vi "AttackerPenalty.vi"(6 "balls":T2[](array[typedef]), 8 "Opponent goalie":T1, 9 "Field Size in":T3, 10 "Numeric":i32, 11 "Robot in":T1) -> (3 "Robot out":T1)   [LabVIEW 2016]
uses:
  Core/AI Robot.ctl
  Core/Field Size.ctl
  Core/AI Ball.ctl
  <vilib>/Analysis/coordinate.llb/Angle Units.ctl
  <vilib>/Analysis/coordinate.llb/Absolute Angle Difference (scalar).vi
  <vilib>/Analysis/coordinate.llb/Wrap Angle (scalar).vi
  <vilib>/Analysis/coordinate.llb/Set Angle Unit.vi
  <vilib>/Analysis/NI_AAL_Angle.lvlib
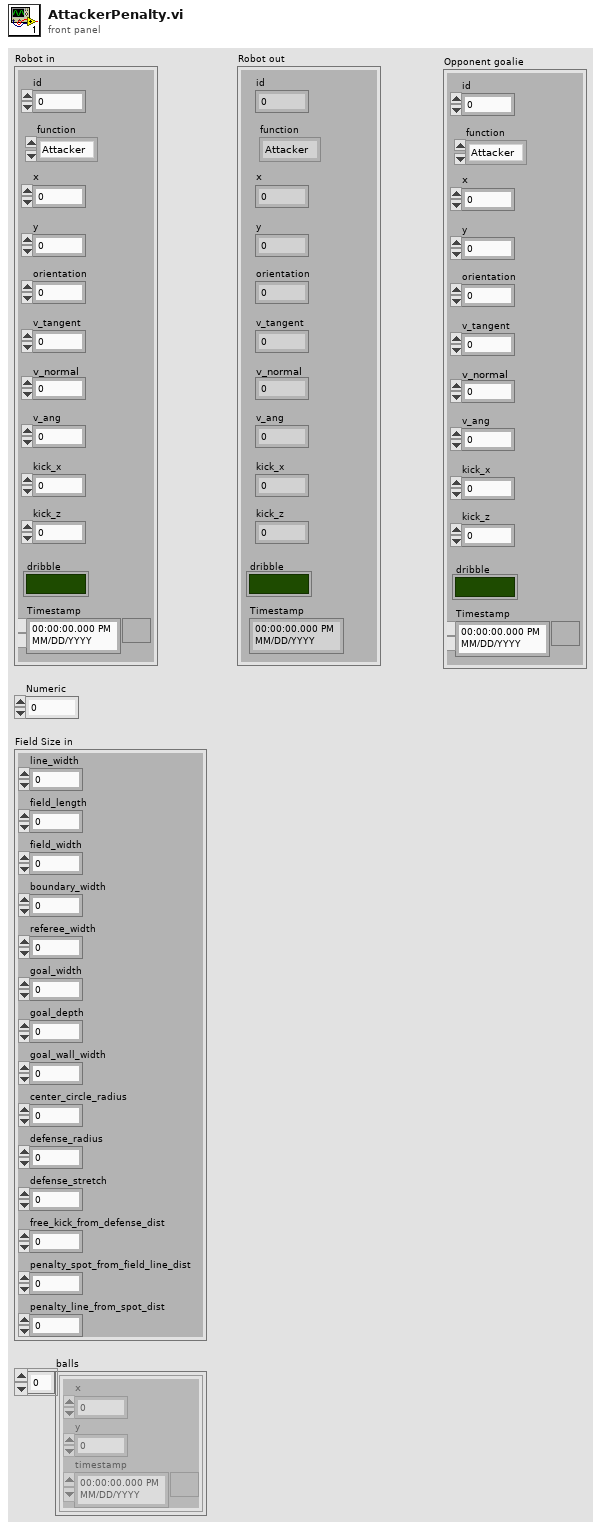
[diagram p1: front panel]
types:
  T1 = typedef "AI Robot.ctl" = cluster{"id":u32, "function":enum16{"Attacker", "Goalie", "Defender"}, "x":dbl, "y":dbl, "orientation":dbl, "v_tangent":dbl, "v_normal":dbl, "v_ang":dbl, "kick_x":dbl, "kick_z":dbl, "dribble":bool, "Timestamp":timestamp}
  T2 = typedef "AI Ball.ctl" = cluster{"x":dbl, "y":dbl, "timestamp":timestamp}
  T3 = typedef "Field Size.ctl" = cluster{"line_width":u32, "field_length":u32, "field_width":u32, "boundary_width":u32, "referee_width":u32, "goal_width":u32, "goal_depth":u32, "goal_wall_width":u32, "center_circle_radius":u32, "defense_radius":u32, "defense_stretch":u32, "free_kick_from_defense_dist":u32, "penalty_spot_from_field_line_dist":u32, "penalty_line_from_spot_dist":u32}
  T4 = typedef "NI_AAL_Angle.lvlib/Angle Units.ctl" = i32
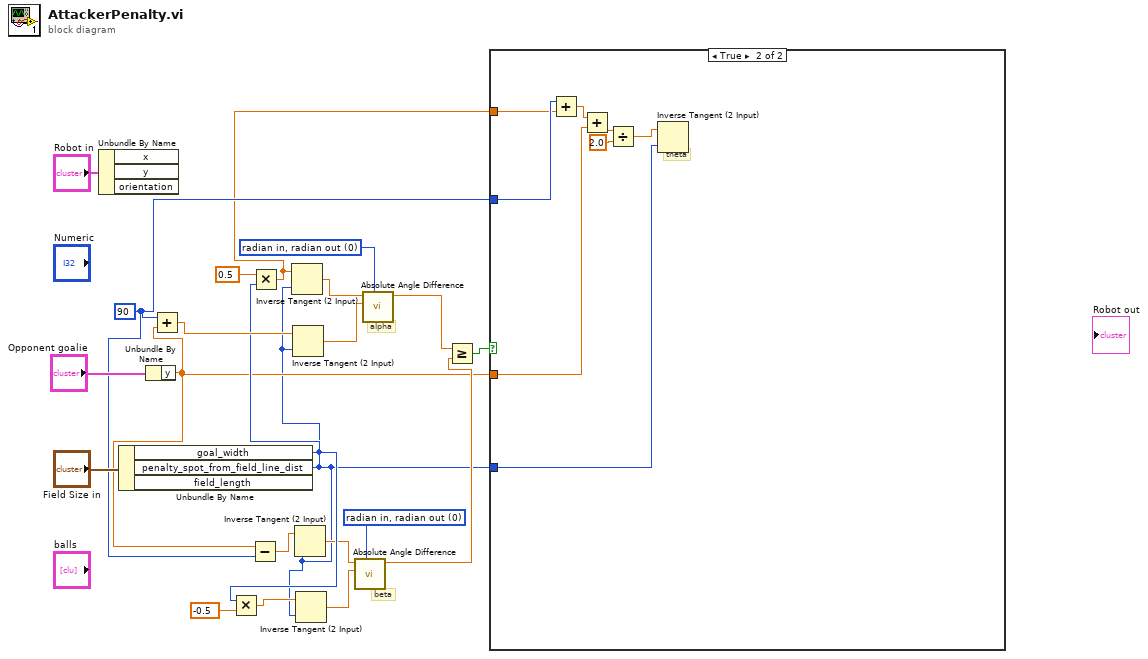
[diagram p0: block diagram]
diagram:
  w8 = T4 0 items=["radian in, radian out", "radian in, degree out", "degree in, degree out", "degree in, radian out"] ("angle units")
  w15 = T4 0 items=["radian in, radian out", "radian in, degree out", "degree in, degree out", "degree in, radian out"] ("angle units")
  w4 = 90
  # "beta"
  # "alpha"
  n1 = Unbundle By Name("Robot in") -> ()  [unwired: 3 out]
  n2 = Unbundle By Name("Field Size in") -> ("goal_width"=w12:u32, "penalty_spot_from_field_line_dist"=w1:u32)  [unwired: 1 out]
  n3 = Unbundle By Name("Opponent goalie") -> ("y"=w2:dbl)
  n4 = Add(x=w4, y=w2) -> (x+y=w20:dbl)
  n5 = Multiply(x=w12, y=-0.5) -> (x*y=w11:dbl)
  n6 = Subtract(x=w2, y=w4) -> (x-y=w14:dbl)
  n7 = Multiply(x=0.5, y=w12) -> (x*y=w3:dbl)
  n8 = Inverse Tangent (2 Input)(1:w1, 2:w3) -> (0:w17:dbl)
  n9 = Inverse Tangent (2 Input)(1:w1, 2:w20) -> (0:w16:dbl)
  n10 = Inverse Tangent (2 Input)(1:w1, 2:w14) -> (0:w10:dbl)
  n11 = Inverse Tangent (2 Input)(1:w1, 2:w11) -> (0:w9:dbl)
  n12 = call-poly <vilib>:"Absolute Angle Difference.vi"("angle units"=w8, "angle 2"=w9, "angle 1"=w10) -> ("absolute angle difference"=w6:dbl)  [unwired: 7 in, 1 out]
  n13 = call-poly <vilib>:"Absolute Angle Difference.vi"("angle units"=w15, "angle 2"=w16, "angle 1"=w17) -> ("absolute angle difference"=w7:dbl)  [unwired: 7 in, 1 out]
  n14 = Greater Or Equal?(x=w7, y=w6) -> (x >= y?=w5:bool)
  n15 = case shown="True" w5 {
    tunnel: w4 -> [_ w30]
    tunnel: w3 -> [_ w29]
    tunnel: w2 -> [_ w27]
    tunnel: w1 -> [_ w23]
    frame False {
    }
    frame True {
      # "theta"
      n16 = Add(x=w30, y=w29) -> (x+y=w28:dbl)
      n17 = Add(x=w28, y=w27) -> (x+y=w25:dbl)
      n18 = Divide(x=w25, y=2.0) -> (x/y=w26:dbl)
      n19 = Inverse Tangent (2 Input)(1:w23, 2:w26) -> ()  [unwired: 1 out]
    }
  }
